vi "TCPReceiver Reset.vi"(8 "error in (no error)":errorcluster, 10 "Flush Buffer (F)":bool, 11 "TCPReceiver in":refnum<class "TCPReceiver.lvclass">) -> (0 "error out":errorcluster, 3 "TCPReceiver out":refnum<class "TCPReceiver.lvclass">)   [LabVIEW 2019, in "TCPReceiver.lvclass"]
uses:
  TCPReceiver.lvclass
  TCPReceiver Progress STYP.ctl
  JSONPacket/JSONPacket.lvclass
  C:/projects/labview_multiplayer_snake_personal/Main Codeline/Software/Code/Shared/TCPPacket/TCPPacket.lvclass
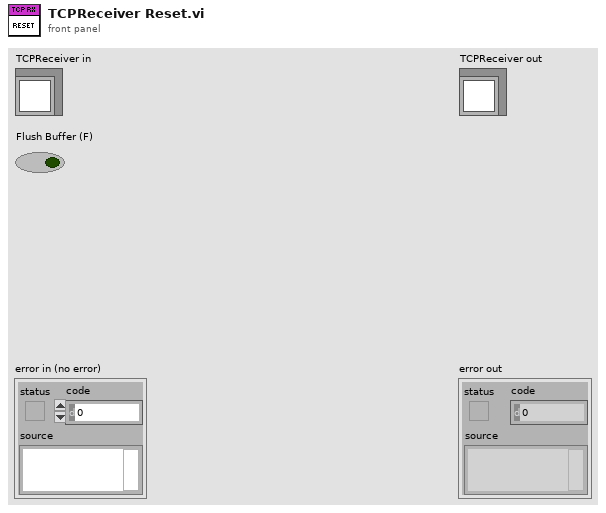
[diagram p1: front panel]
types:
  T1 = typedef "TCPReceiver.lvclass/TCPReceiver Progress STYP.ctl" = cluster{"HeaderSize?":bool, "Header?":bool, "Body?":bool}
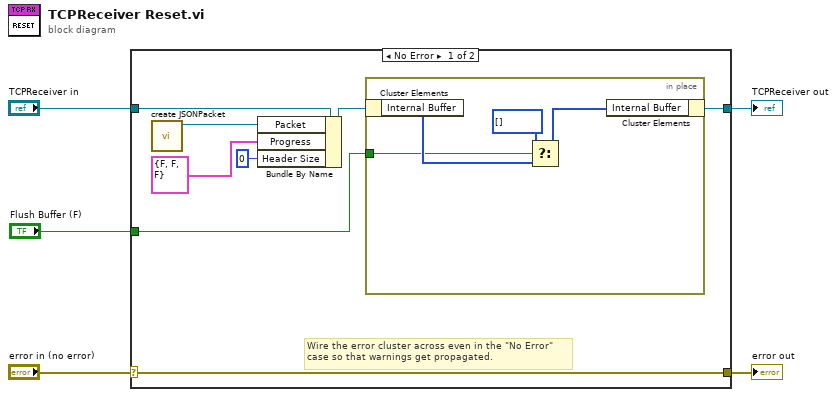
[diagram p0: block diagram]
diagram:
  n1 = case shown="No Error" "error in (no error)" {
    selector: "error in (no error)" -> [w12 w19]
    tunnel: [w12 w19] -> w4
    tunnel: [w7 w18] -> w2
    tunnel: "TCPReceiver in" -> [w13 w18]
    tunnel: "Flush Buffer (F)" -> [w6 _]
    frame No Error {
      # "Wire the error cluster across even in the \"No Error\"\ncase so that warnings get propagated."
      n2 = call "create JSONPacket.vi"() -> ("JSONPacket out"=w9:refnum<class "JSONPacket.lvclass">)  [unwired: 10 in, 1 out]
      n3 = Bundle By Name(cluster=w13, "Packet"=w9, "Progress"=T1 {"HeaderSize?"=FALSE, "Header?"=FALSE, "Body?"=FALSE}, "Header Size"=u16 0) -> (w8:refnum<class "TCPReceiver.lvclass">)
      n4 = in-place {
        in-place-border: w6 -> [w15]
        n5 = in-place-cluster #1(w8) -> ("Internal Buffer"=w17:u8[])
        n6 = Select(t=u8[] [], s=w15, f=w17) -> (s? t:f=w16:u8[])
        n7 = in-place-cluster #1("Internal Buffer"=w16) -> (w7:refnum<class "TCPReceiver.lvclass">)
      }
    }
    frame Error {
    }
  }
  "error out" <- w4
  "TCPReceiver out" <- w2
